vi "Scale.vi"(8 "error in (no error)":errorcluster, 10 "Scale Factor":dbl, 11 "Collection in":refnum<class "Collection.lvclass">) -> (0 "error out":errorcluster, 3 "Collection out":refnum<class "Collection.lvclass">)   [LabVIEW 2021, in "Picture2D.lvlib" / "Collection.lvclass"]
uses:
  Collection.lvclass
  Collection.lvclass/Collection.ctl
  IDrawable/IDrawable.lvclass
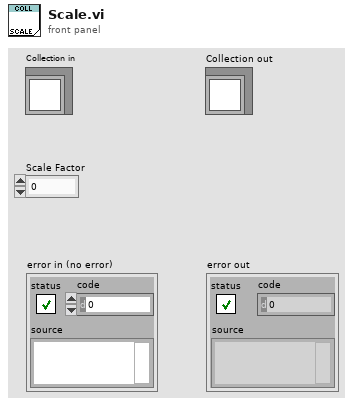
[diagram p1: front panel]
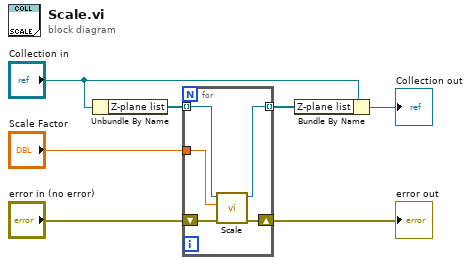
[diagram p0: block diagram]
diagram:
  n1 = Unbundle By Name("Collection in") -> ("Z-plane list"=w5:refnum<class "IDrawable.lvclass">[])
  n2 = for {
    tunnel: w5 -> [w12] mode=indexing
    tunnel: [w11] -> w4 mode=indexing
    tunnel: "Scale Factor" -> [w10]
    shift-right: [w8] -> w1
    shift-left: "error in (no error)" -> [w9]
    n3 = call-dynamic "Scale.vi"("error in (no error)"=w9, "Scale Factor"=w10, "IScalable in"=w12) -> ("error out"=w8:errorcluster, "IScalable out"=w11:refnum<class "IDrawable.lvclass">)  [unwired: 7 in]
  }
  "error out" <- w1
  n4 = Bundle By Name(cluster="Collection in", "Z-plane list"=w4) -> (→"Collection out":refnum<class "Collection.lvclass">)
